vi "addNewAction.vi"(8 "error in (no error)":errorcluster, 10 "newAction":string, 11 "Log in":refnum<class "Log.lvclass">) -> (0 "error out":errorcluster, 3 "Log out":refnum<class "Log.lvclass">)   [LabVIEW 2009, in "Tools.lvlib" / "xml.lvlib" / "Log.lvclass"]
uses:
  Log.lvclass
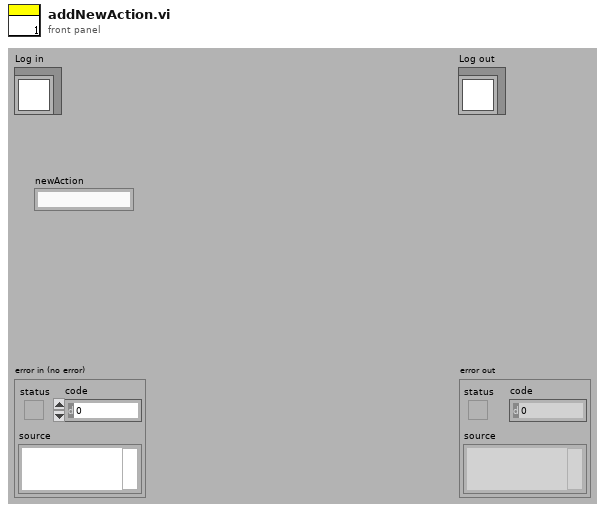
[diagram p1: front panel]
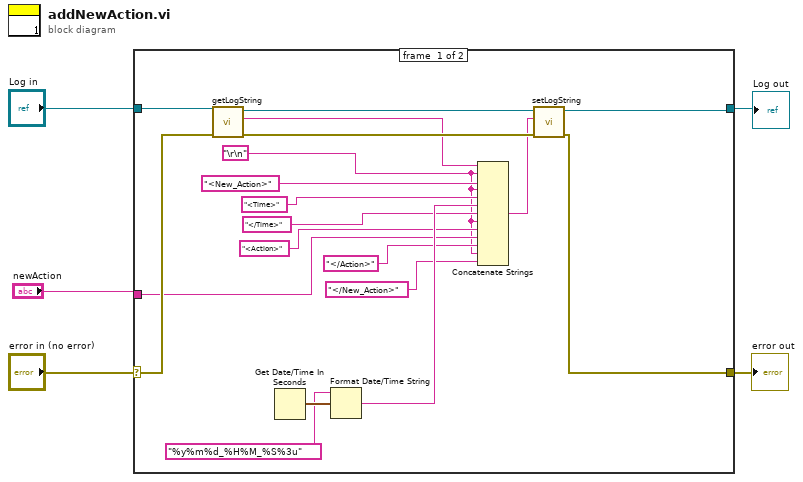
[diagram p0: block diagram]
diagram:
  n1 = case shown="No Error" "error in (no error)" {
    selector: "error in (no error)" -> [w23 w26]
    tunnel: [w20 w26] -> w4
    tunnel: [w19 w25] -> w2
    tunnel: "Log in" -> [w24 w25]
    tunnel: "newAction" -> [w9 _]
    frame #0 {
      w7 = "\r\n"
      n2 = call-dynamic "getLogString.vi"("error in (no error)"=w23, "Log.lvclass in"=w24) -> ("error out"=w21:errorcluster, "logString"=w14:string, "Log.lvclass out"=w22:refnum<class "Log.lvclass">)  [unwired: 7 in]
      n3 = Get Date/Time In Seconds() -> (seconds since 1Jan1904=w18:timestamp)
      n4 = Format Date/Time String(time format string (%c)="%y%m%d_%H%M_%S%3u", seconds (now)=w18) -> (date/time string=w12:string)  [unwired: 1 in]
      n5 = Concatenate Strings(w14, w7, "<New_Action>", w7, "<Time>", w12, "</Time>", w7, "<Action>", w9, "</Action>", w7, "</New_Action>") -> (w16:string)
      n6 = call-dynamic "setLogString.vi"("error in (no error)"=w21, "logString"=w16, "Log.lvclass in"=w22) -> ("error out"=w20:errorcluster, "Log.lvclass out"=w19:refnum<class "Log.lvclass">)  [unwired: 7 in]
    }
    frame #1 {
    }
  }
  "error out" <- w4
  "Log out" <- w2
